vi "Untitled 1.vi"() -> ()   [LabVIEW 2015]
panel:
  out "refnum out":refnum<file>
  out "cancelled":bool
  out "error out":errorcluster
  out "text":string
  out "array":string[](array[string])
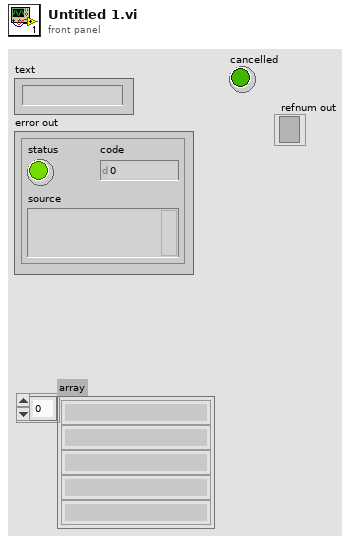
[diagram p1: front panel]
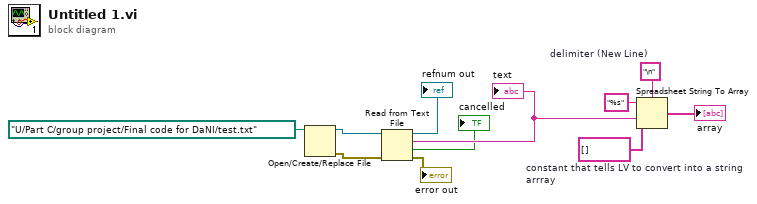
[diagram p0: block diagram]
diagram:
  w8 = "\n"  # delimiter (New Line)
  w11 = string[] []  # constant that tells LV to convert into a string arrray
  n1 = Open/Create/Replace File(file path (use dialog)=path "U:/Part C/group project/Final code for DaNI/test.txt") -> (refnum out=w6:refnum<file>, error out=w5:errorcluster)  [unwired: 5 in, 1 out]
  n2 = Read from Text File(file (use dialog)=w6, error in=w5) -> (refnum out=→"refnum out":refnum<file>, text=w4:string, cancelled=→"cancelled":bool, error out=→"error out":errorcluster)  [unwired: 2 in]
  "text" <- w4
  n3 = Spreadsheet String To Array(delimiter (Tab)=w8, format string="%s", spreadsheet string=w4, array type (2D Dbl)=w11) -> (array=→"array":string[])
